vi "Initial7230.vi"(8 "error in (no error)":errorcluster caption="错误输入（无错误）") -> (0 "error out":errorcluster caption="错误输出", 1 "task out Output":refnum<k7>, 3 "task out Input":refnum<k7>)   [LabVIEW 2017]
uses:
  <userlib>/DAQPilot/create/channels.llb/PLT Create Channel (DI-Digital Input).vi
  <userlib>/DAQPilot/create/channels.llb/PLT Create Channel (DO-Digital Output).vi
panel:
  in  "lines 2":string="Dev0/Port0/line0:15"
  in  "lines":string="Dev0/port0/Line0:15"
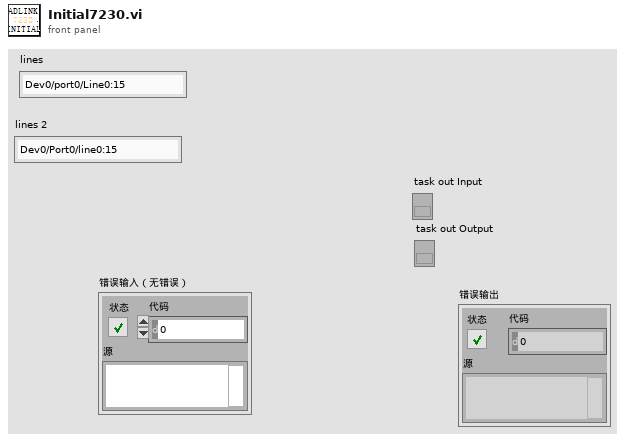
[diagram p1: front panel]
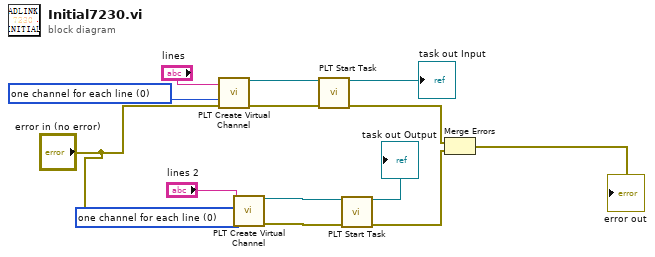
[diagram p0: block diagram]
diagram:
  w8 = 0 items=["one channel for each line", "one channel for all lines"] ("line grouping")
  w14 = 0 items=["one channel for each line", "one channel for all lines"] ("line grouping")
  n1 = call-poly <userlib>:"PLT Create Virtual Channel.vi"("lines"="lines", "line grouping"=w14, "error in"="error in (no error)") -> ("task out"=w12:refnum<k7>, "error out"=w11:errorcluster)  [unwired: 11 in]
  n2 = call-poly <userlib>:"PLT Create Virtual Channel.vi"("lines"="lines 2", "line grouping"=w8, "error in"="error in (no error)") -> ("task out"=w10:refnum<k7>, "error out"=w9:errorcluster)  [unwired: 11 in]
  n3 = call <userlib>:"PLT Start Task.vi"("task/channels in"=w12, "error in"=w11) -> ("task out"=→"task out Input":refnum<k7>, "error out"=w5:errorcluster)  [unwired: 12 in]
  n4 = call <userlib>:"PLT Start Task.vi"("task/channels in"=w10, "error in"=w9) -> ("task out"=→"task out Output":refnum<k7>, "error out"=w4:errorcluster)  [unwired: 12 in]
  n5 = Merge Errors(w5, w4) -> (→"error out":errorcluster)
